vi "Global_SSC.vi"(8 "Error In":errorcluster, 9 "Write?":bool, 11 "SSC In (meters)":dbl[](array[numeric]) format="%_6g") -> (0 "Error Out":errorcluster, 3 "SSC Out (meters)":dbl[](array[numeric]) format="%_6g")   [LabVIEW 2019]
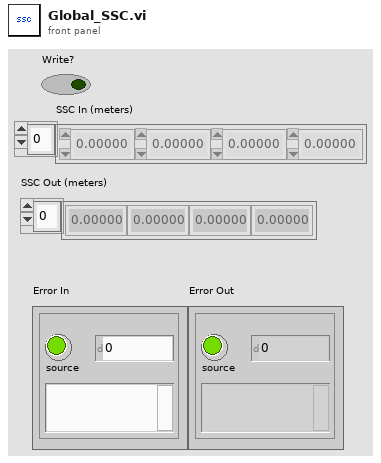
[diagram p1: front panel]
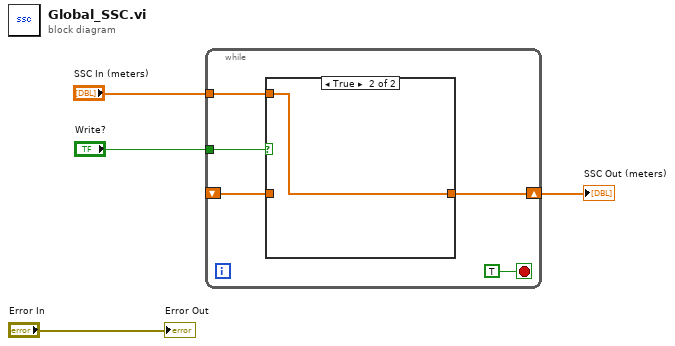
[diagram p0: block diagram]
diagram:
  n1 = while {
    tunnel: "Write?" -> [w9]
    shift-right: [w7] -> w3
    shift-left: _ -> [w5]
    tunnel: "SSC In (meters)" -> [w6]
    stop <- TRUE stop-if-true
    n2 = case shown="True" w9 {
      tunnel: [w10 w11] -> w7
      tunnel: w6 -> [_ w11]
      tunnel: w5 -> [w10 _]
      frame False {
      }
      frame True {
      }
    }
  }
  "SSC Out (meters)" <- w3
  "Error Out" <- "Error In"
